vi "LogModbusEvent.vi"(0 "reference in":refnum<class "Stand.lvclass">, 5 "Data Read":T1, 11 "error in (no error)":errorcluster) -> (4 "reference out":refnum<class "Stand.lvclass">, 15 "error out":errorcluster)   [LabVIEW 2019, in "Stand.lvclass"]
uses:
  Stand.lvclass
  Modbus_class/ReadData.ctl
  Stand.lvclass/Stand.ctl
  AI_class/AI.lvclass/AI.ctl
  PiecedLinearScale_class/Scale_PiecedLinear.lvclass/Scale_PiecedLinear.ctl
  Proccess_class/Proccess.lvclass/Proccess.ctl
  Logger_class/Logger.lvclass/Logger.ctl
  AnalogComparator_class/AnalogComparator.lvclass/AnalogComparator.ctl
  PiecedLinearScale_class/RawToScaled.vi
  subvis/Average.vi
  subvis/Loop Time Const.vi
  AI_class/HandleRanges.vi
  AI_class/HandleAlarms.vi
  AI_class/private/WriteToDb.vi
  AnalogComparator_class/SetValue.vi
  Logger_class/Enqueue Signal.vi
  AI_class/AI.lvclass
  C:/Users/ANENKOV_V1/Desktop/src/Proccess_class/Proccess.lvclass
  <vilib>/gmath/interp.llb/Interpolate 1D.vi
  <vilib>/Utility/error.llb/Error Cluster From Error Code.vi
  AnalogComparator_class/SendToDb.vi
  Proccess_class/Proccess.lvclass
  Logger_class/Logger.lvclass
  TypeDef/MB CMD.ctl
  TypeDef/AlarmType.ctl
  Logger_class/EventData.ctl
  a68f8bf2-9450-45a9-b6c2-f7836ab310e2.vi
  Modbus_class/ModbusSp.lvclass
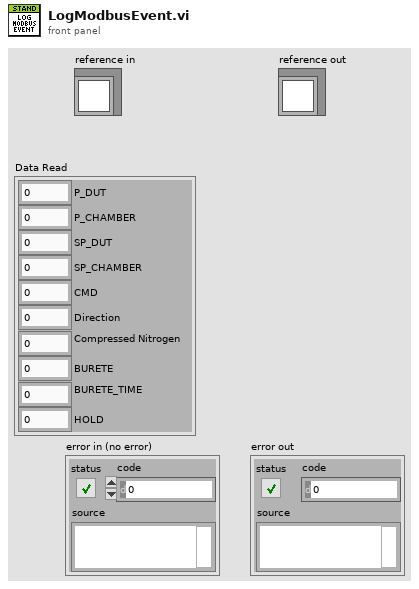
[diagram p1: front panel]
types:
  T1 = typedef "ModbusSp.lvclass/ReadData.ctl" = cluster{"P_DUT":sgl, "P_CHAMBER":sgl, "SP_DUT":sgl, "SP_CHAMBER":sgl, "CMD":u16, "Direction":u16, "Compressed Nitrogen":u16, "BURETE":u16, "BURETE_TIME":u16, "HOLD":u16}
  T2 = typedef "MB CMD.ctl" = cluster{"START":bool, "PRESS_DOWN_SLOW":bool}
  T3 = typedef "AlarmType.ctl" = enum16{"Normal", "Warning", "Alarm"}
  T4 = typedef "EventData.ctl" = cluster{"obj_tag":string, "event_tag":string, "Description":string, "ALARM TYPE":T3, "Value DBL":dbl, "Value INT":i32, "Value STR":string, "Time Stamp":timestamp}
  T5 = cluster{"Boolean array[0]":bool, "Boolean array[1]":bool}
  T6 = typedef "Proccess.lvclass/TAGs.ctl" = cluster{"TAG":string, "PTAG":string, "DESC":string}
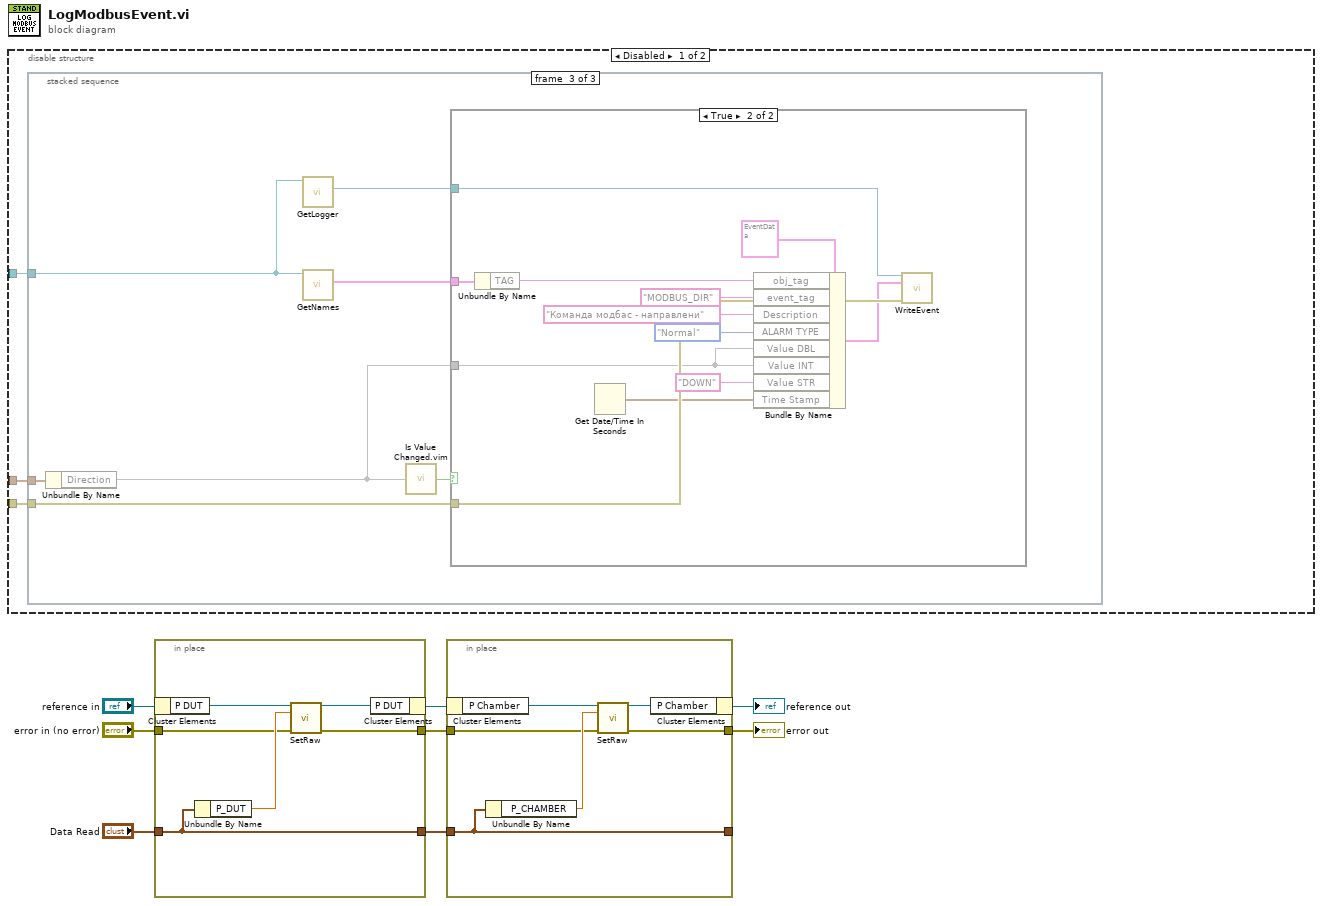
[diagram p0: block diagram]
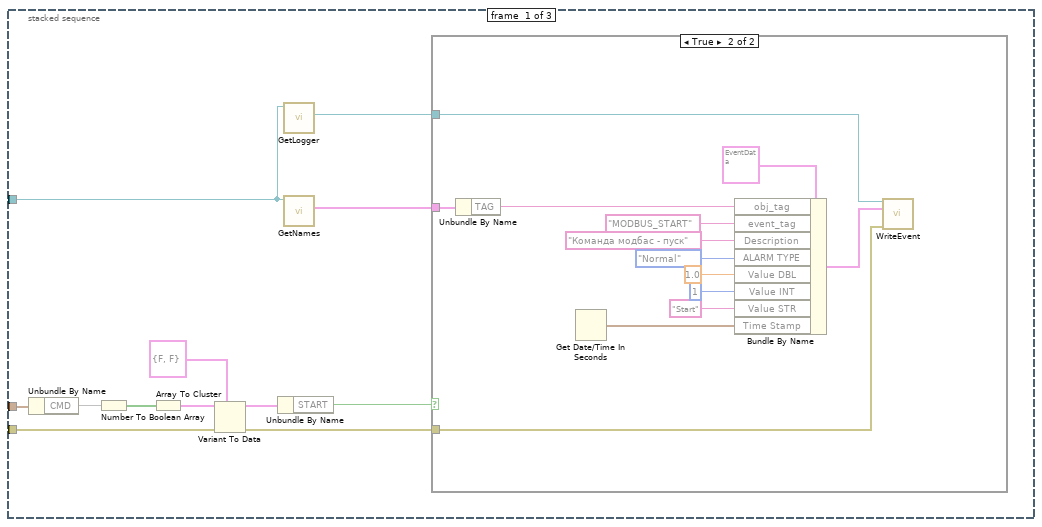
[diagram p2: hidden frame]
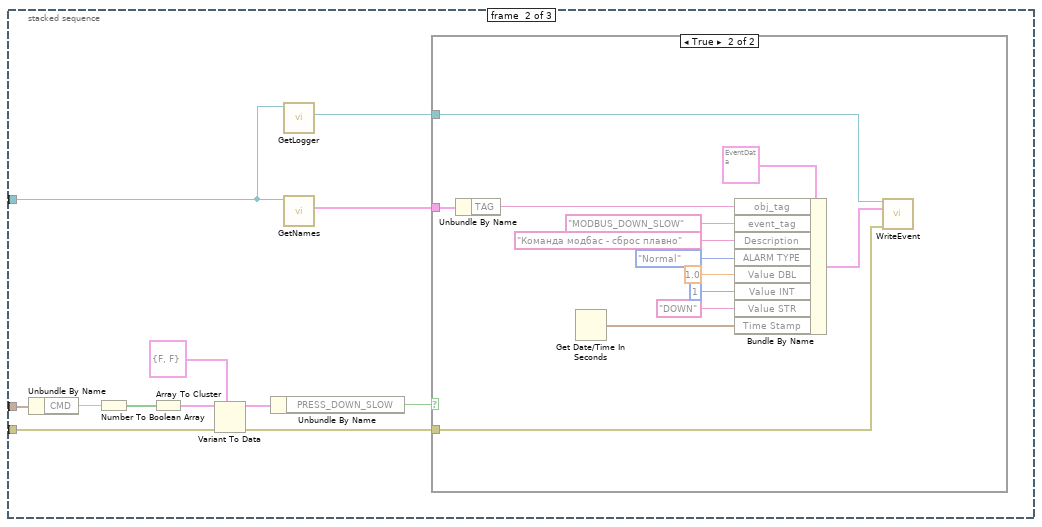
[diagram p4: hidden frame]
diagram:
  n1 = disable-structure shown="Disabled" {
    disable-tunnel: _ -> [w11 _]
    disable-tunnel: _ -> [w10 _]
    disable-tunnel: _ -> [w9 _]
    frame Disabled {
      n2 = stacked-sequence {
        tunnel: w11 -> [w23 w48 w68]
        tunnel: w10 -> [w18 w43 w67]
        tunnel: w9 -> [w13 w38 w65]
        frame #0 {
          n3 = Unbundle By Name(w23) -> ("CMD"=w22)
          n4 = Number To Boolean Array(number=w22) -> (Boolean array=w21:bool[])
          n5 = Array To Cluster(array=w21) -> (cluster=w20:T5)
          n6 = Variant To Data(error in=w18, type=T2 {"START"=FALSE, "PRESS_DOWN_SLOW"=FALSE} ("MB CMD"), Variant=w20) -> (data=w17:T2, error out=w14:errorcluster)
          n7 = Unbundle By Name(w17) -> ("START"=w16:bool)
          n8 = call "GetLogger.vi"("Proccess in"=w13) -> ("Logger"=w15:refnum<class "Logger.lvclass">)  [unwired: 10 in]
          n9 = call "GetNames.vi"("Proccess in"=w13) -> ("Tags"=w12:T6)  [unwired: 10 in]
          n10 = case shown="True" w16 {
            tunnel: w15 -> [_ w36]
            tunnel: w14 -> [_ w34]
            tunnel: w12 -> [_ w32]
            frame False {
            }
            frame True {
              n11 = Unbundle By Name(w32) -> ("TAG"=w31:string)
              n12 = Get Date/Time In Seconds() -> (seconds since 1Jan1904=w24:timestamp)
              n13 = Bundle By Name(cluster=T4 {"obj_tag"="", "event_tag"="", "Description"="", "ALARM TYPE"=enum."Alarm", "Value DBL"=0.0, "Value INT"=0, "Value STR"="", "Time Stamp"=timestamp(0 s since 1904-01-01)} ("Event"), "obj_tag"=w31, "event_tag"="MODBUS_START", "Description"="Команда модбас - пуск", "ALARM TYPE"=AlarmType."Normal", "Value DBL"=1.0, "Value INT"=1, "Value STR"="Start", "Time Stamp"=w24) -> (w33:T4)
              n14 = call "WriteEvent.vi"("reference in"=w36, "Event"=w33, "error in (no error)"=w34) -> ()  [unwired: 11 in, 2 out]
            }
          }
        }
        frame #1 {
          n15 = Unbundle By Name(w48) -> ("CMD"=w47)
          n16 = Number To Boolean Array(number=w47) -> (Boolean array=w46:bool[])
          n17 = Array To Cluster(array=w46) -> (cluster=w45:T5)
          n18 = Variant To Data(error in=w43, type=T2 {"START"=FALSE, "PRESS_DOWN_SLOW"=FALSE} ("MB CMD"), Variant=w45) -> (data=w42:T2, error out=w39:errorcluster)
          n19 = Unbundle By Name(w42) -> ("PRESS_DOWN_SLOW"=w41:bool)
          n20 = call "GetLogger.vi"("Proccess in"=w38) -> ("Logger"=w40:refnum<class "Logger.lvclass">)  [unwired: 10 in]
          n21 = call "GetNames.vi"("Proccess in"=w38) -> ("Tags"=w37:T6)  [unwired: 10 in]
          n22 = case shown="True" w41 {
            tunnel: w40 -> [_ w61]
            tunnel: w39 -> [_ w59]
            tunnel: w37 -> [_ w57]
            frame False {
            }
            frame True {
              n23 = Unbundle By Name(w57) -> ("TAG"=w56:string)
              n24 = Get Date/Time In Seconds() -> (seconds since 1Jan1904=w49:timestamp)
              n25 = Bundle By Name(cluster=T4 {"obj_tag"="", "event_tag"="", "Description"="", "ALARM TYPE"=enum."Alarm", "Value DBL"=0.0, "Value INT"=0, "Value STR"="", "Time Stamp"=timestamp(0 s since 1904-01-01)} ("Event"), "obj_tag"=w56, "event_tag"="MODBUS_DOWN_SLOW", "Description"="Команда модбас - сброс плавно", "ALARM TYPE"=AlarmType."Normal", "Value DBL"=1.0, "Value INT"=1, "Value STR"="DOWN", "Time Stamp"=w49) -> (w58:T4)
              n26 = call "WriteEvent.vi"("reference in"=w61, "Event"=w58, "error in (no error)"=w59) -> ()  [unwired: 11 in, 2 out]
            }
          }
        }
        frame #2 {
          n27 = Unbundle By Name(w68) -> ("Direction"=w62)
          n28 = call "GetLogger.vi"("Proccess in"=w65) -> ("Logger"=w66:refnum<class "Logger.lvclass">)  [unwired: 10 in]
          n29 = call "GetNames.vi"("Proccess in"=w65) -> ("Tags"=w64:T6)  [unwired: 10 in]
          n30 = call "Is Value Changed.vim"("value"=w62) -> ("changed or first call?"=w63:bool)
          n31 = case shown="True" w63 {
            tunnel: w66 -> [_ w80]
            tunnel: w67 -> [_ w78]
            tunnel: w64 -> [_ w76]
            tunnel: w62 -> [_ w69]
            frame False {
            }
            frame True {
              n32 = Unbundle By Name(w76) -> ("TAG"=w75:string)
              n33 = Get Date/Time In Seconds() -> (seconds since 1Jan1904=w70:timestamp)
              n34 = Bundle By Name(cluster=T4 {"obj_tag"="", "event_tag"="", "Description"="", "ALARM TYPE"=enum."Alarm", "Value DBL"=0.0, "Value INT"=0, "Value STR"="", "Time Stamp"=timestamp(0 s since 1904-01-01)} ("Event"), "obj_tag"=w75, "event_tag"="MODBUS_DIR", "Description"="Команда модбас - направлени", "ALARM TYPE"=AlarmType."Normal", "Value DBL"=w69, "Value INT"=w69, "Value STR"="DOWN", "Time Stamp"=w70) -> (w77:T4)
              n35 = call "WriteEvent.vi"("reference in"=w80, "Event"=w77, "error in (no error)"=w78) -> ()  [unwired: 11 in, 2 out]
            }
          }
        }
      }
    }
    frame Enabled {
    }
  }
  n36 = in-place {
    in-place-border: "Data Read" -> [w84]
    in-place-border: [w84] -> w3
    in-place-border: "error in (no error)" -> [w82]
    in-place-border: [w81] -> w4
    n37 = in-place-cluster #1("reference in") -> ("P DUT"=w86:refnum<class "AI.lvclass">)
    n38 = Unbundle By Name(w84) -> ("P_DUT"=w83:sgl)
    n39 = call "SetRaw.vi"("reference in"=w86, "raw mean"=w83, "error in (no error)"=w82) -> ("reference out"=w85:refnum<class "AI.lvclass">, "error out"=w81:errorcluster)  [unwired: 11 in]
    n40 = in-place-cluster #1("P DUT"=w85) -> (w5:refnum<class "Stand.lvclass">)
  }
  n41 = in-place {
    in-place-border: w3 -> [w90]
    in-place-border: [w90] -> _
    in-place-border: w4 -> [w88]
    in-place-border: [w87] -> w1
    n42 = in-place-cluster #2(w5) -> ("P Chamber"=w92:refnum<class "AI.lvclass">)
    n43 = Unbundle By Name(w90) -> ("P_CHAMBER"=w89:sgl)
    n44 = call "SetRaw.vi"("reference in"=w92, "raw mean"=w89, "error in (no error)"=w88) -> ("reference out"=w91:refnum<class "AI.lvclass">, "error out"=w87:errorcluster)  [unwired: 11 in]
    n45 = in-place-cluster #2("P Chamber"=w91) -> (→"reference out":refnum<class "Stand.lvclass">)
  }
  "error out" <- w1
